vi "Add Status to Tree.vi"(6 "Show Metrics":bool, 8 "error in":errorcluster, 10 "Status Tree":map{string[], T1}(c390), 11 "Tree Map in":refnum<class "Tree Map.lvclass">) -> (0 "error out":errorcluster, 3 "Tree Map":refnum<class "Tree Map.lvclass">)   [LabVIEW 2020, in "VolatusGUI.lvlib" / "Debug GUI Module.lvclass"]
uses:
  Debug GUI Module.lvclass
  Debug GUI Module.lvclass/Debug GUI Module.ctl
  lv-tree-tools/Tree Map/Tree Map/Tree Map.lvclass
  lv-tree-tools/Tree Map/Tree Map/Extra Entry Info.ctl
  Volatus/Module/State.ctl
  Volatus/Module/Module.lvclass
  Volatus/Module Status.ctl
  Volatus/Volatus.lvlib
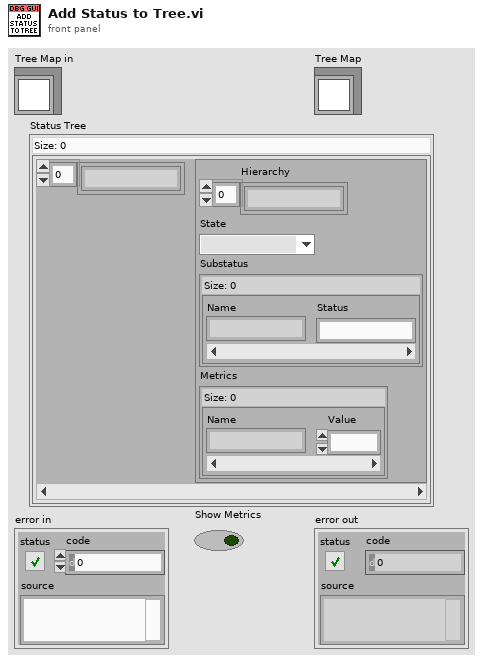
[diagram p1: front panel]
types:
  T1 = typedef "Volatus.lvlib/Module Status.ctl" = cluster{"Hierarchy":string[], "State":T2, "Substatus":map{string, string}, "Metrics":map{string, dbl}}
  T2 = typedef "Volatus.lvlib/Module.lvclass/State.ctl" = enum16{"Unknown", "Launched", "Starting", "Running", "Stopping", "Stopped", "Error - Starting", "Error - Run", "Error - Stopping"}
  T3 = typedef "Tree Map.lvlib/Tree Map.lvclass/Extra Entry Info.ctl" = cluster{"BG Color":u32, "Symbol":i32}
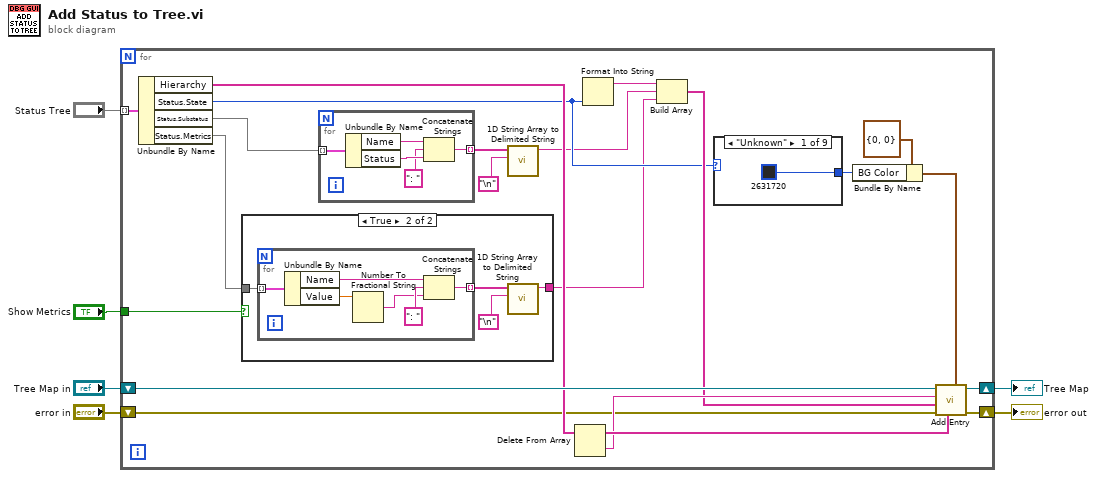
[diagram p0: block diagram]
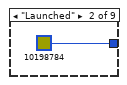
[diagram p3: hidden frame]
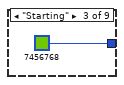
[diagram p4: hidden frame]
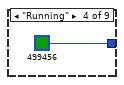
[diagram p5: hidden frame]
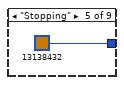
[diagram p6: hidden frame]
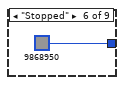
[diagram p7: hidden frame]
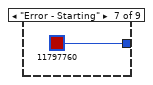
[diagram p8: hidden frame]
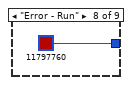
[diagram p9: hidden frame]
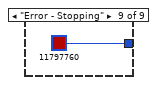
[diagram p10: hidden frame]
diagram:
  n1 = for {
    tunnel: "Status Tree" -> [w27] mode=indexing
    shift-right: [w22] -> w4
    shift-left: "Tree Map in" -> [w26]
    shift-right: [w18] -> w3
    shift-left: "error in" -> [w19]
    tunnel: "Show Metrics" -> [w10]
    n2 = Unbundle By Name(w27) -> ("Hierarchy"=w25:string[], "Status.State"=w17:T2, "Status.Substatus"=w16:map{string, string}, "Status.Metrics"=w12:map{string, dbl})
    n3 = case shown="True" w10 {
      tunnel: w12 -> [_ w29]
      tunnel: [_ w28] -> w11
      frame False {
      }
      frame True {
        n4 = for {
          tunnel: w29 -> [w37] mode=indexing
          tunnel: [w34] -> w30 mode=indexing
          n5 = Unbundle By Name(w37) -> ("Name"=w36:string, "Value"=w33:dbl)
          n6 = Number To Fractional String(number=w33) -> (F-format string=w32:string)  [unwired: 3 in]
          n7 = Concatenate Strings(w36, ": ", w32) -> (w34:string)
        }
        n8 = call <vilib>:"1D String Array to Delimited String.vi"("delimiter"="\n", "string array"=w30) -> ("delimited string"=w28:string)  [unwired: 9 in]
      }
    }
    n9 = for {
      tunnel: w16 -> [w42] mode=indexing
      tunnel: [w38] -> w15 mode=indexing
      n10 = Unbundle By Name(w42) -> ("Name"=w41:string, "Status"=w40:string)
      n11 = Concatenate Strings(w41, ": ", w40) -> (w38:string)
    }
    n12 = call <vilib>:"1D String Array to Delimited String.vi"("delimiter"="\n", "string array"=w15) -> ("delimited string"=w13:string)  [unwired: 9 in]
    n13 = Delete From Array(array=w25) -> (deleted portion=w23:string, array with subset deleted=w24:string[])  [unwired: 2 in]
    n14 = Format Into String(w17) -> (resulting string=w21:string)  [unwired: 3 in, 1 out]
    n15 = Build Array(w21, w13, w11) -> (w20:string[])
    n16 = case shown="\"Unknown\"" w17 {
      tunnel: [u32 2631720 u32 10198784 u32 7456768 u32 499456 u32 13138432 u32 9868950 u32 11797760 u32 11797760 u32 11797760] -> w9
      frame "Unknown" {
      }
      frame "Launched" {
      }
      frame "Starting" {
      }
      frame "Running" {
      }
      frame "Stopping" {
      }
      frame "Stopped" {
      }
      frame "Error - Starting" {
      }
      frame "Error - Run" {
      }
      frame "Error - Stopping" {
      }
    }
    n17 = Bundle By Name(cluster=T3 {"BG Color"=0, "Symbol"=0} ("Extra Info"), "BG Color"=w9) -> (w7:T3)
    n18 = call "Add Entry.vi"("Extra Info"=w7, "Parent (None)"=w24, "error in (no error)"=w19, "Columns"=w20, "Name"=w23, "Tree Map in"=w26) -> ("error out"=w18:errorcluster, "Tree Map out"=w22:refnum<class "Tree Map.lvclass">)  [unwired: 3 in, 1 out]
  }
  "Tree Map" <- w4
  "error out" <- w3
